vi "qr.vi"(9 "stop":bool, 11 "Session In":T2) -> (1 "Image":T1(plugin-control), 2 "Found?":bool, 3 "Data":string)   [LabVIEW 2019]
uses:
  <vilib>/userdefined/High Color/IMAQdx.ctl
  <vilib>/vision/driver/NI_Vision_Acquisition_Software.lvlib
  <vilib>/vision/NI_Vision_Development_Module.lvlib
panel:
  out "error out 2":errorcluster
  out "error out 3":errorcluster
  out "error out":errorcluster
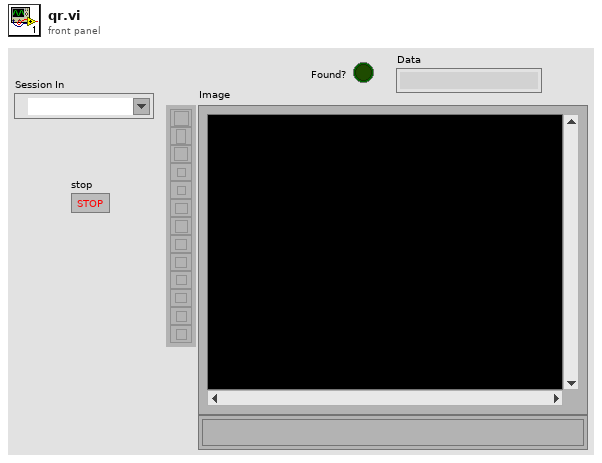
[diagram p1: front panel]
types:
  T1 = typedef "IMAQ Image.ctl" = refnum<image>
  T2 = typedef "IMAQdx.ctl" = refnum<k21>
  T3 = typedef "Image Type" = u32
  T4 = typedef "QR Code Report.ctl" = cluster{"Found?":bool, "Data":string, "Bounding Box":cluster{"x":sgl, "y":sgl}[], "Errors Corrected":u32, "Dimensions (Rows/Cols)":u32, "Version":u32, "QR Model":T5, "Stream Mode":T6, "Barcode Polarity":T7, "Mirrored?":bool, "Append Stream Position":u32, "Size of Append Stream":u32, "First EAN-128 ID":i32, "First Alternate Language ID":i32, "Append Stream ID":u32, "Minimum Edge Strength":u32, "Demodulation Mode":T8, "Cell Sample Size":T9, "Cell Filter Mode":T10}
  T5 = typedef "QR Code Model Type.ctl" = i32
  T6 = typedef "QR Code Stream Mode Type.ctl" = i32
  T7 = typedef "Data Matrix Polarity.ctl" = i32
  T8 = typedef "Demodulation Mode.ctl" = i32
  T9 = typedef "Cell Sample Size.ctl" = i32
  T10 = typedef "Cell Filter Mode.ctl" = i32
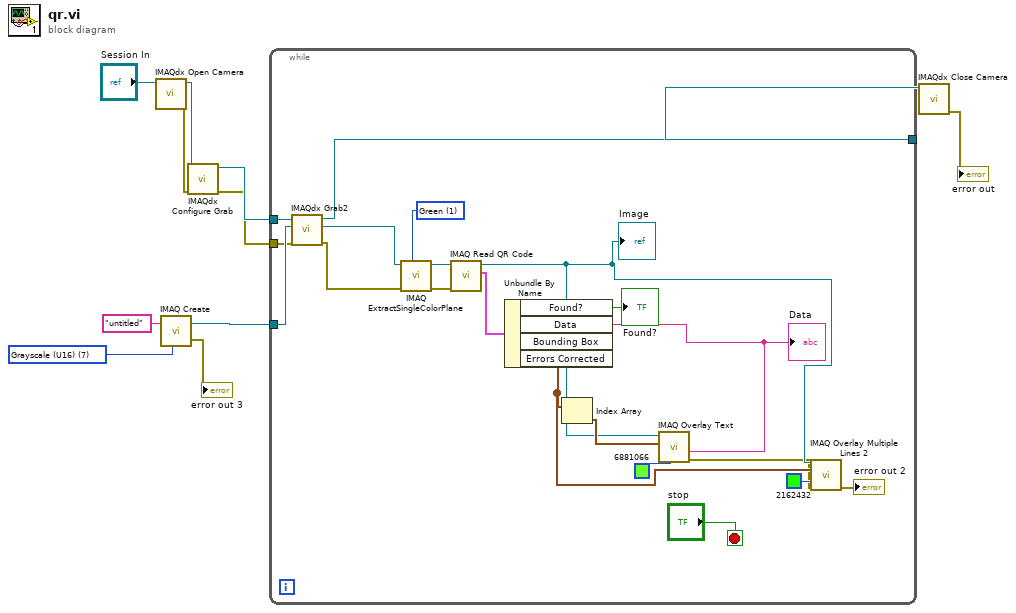
[diagram p0: block diagram]
diagram:
  w1 = T3 7 items=["Grayscale (U8)", "Grayscale (I16)", "Grayscale (SGL)", "Complex (CSG)", "RGB (U32)", "HSL (U32)", "RGB (U64)", "Grayscale (U16)"] ("Image Type")
  n1 = call <vilib>:"IMAQdx Open Camera.vi"("Session In"="Session In") -> ("error out"=w9:errorcluster, "Session Out"=w10:T2)  [unwired: 9 in]
  n2 = call "IMAQ Create"("Image Name"="untitled", "Image Type"=w1) -> ("New Image"=w6:T1, "error out"=→"error out 3":errorcluster)  [unwired: 3 in]
  n3 = call <vilib>:"IMAQdx Configure Grab.vi"("error in"=w9, "Session In"=w10) -> ("error out"=w3:errorcluster, "Session Out"=w7:T2)  [unwired: 8 in]
  n4 = while {
    tunnel: w7 -> [w30]
    tunnel: w6 -> [w31]
    tunnel: [w23] -> w4
    tunnel: w3 -> [w28]
    stop <- "stop" stop-if-true
    w22 = 1 items=["Red", "Green", "Blue", "Hue", "Saturation", "Luminance", "Value", "Intensity"] ("Color Plane")
    n5 = call <vilib>:"IMAQdx Grab2.vi"("error in"=w28, "Image In"=w31, "Session In"=w30) -> ("error out"=w25:errorcluster, "Image Out"=w24:T1, "Session Out"=w23:T2)  [unwired: 5 in, 1 out]
    n6 = call "IMAQ ExtractSingleColorPlane"("Color Plane"=w22, "error in (no error)"=w25, "Image Src"=w24) -> ("error out"=w27:errorcluster, "Image Dst Out"=w26:T1)  [unwired: 7 in]
    n7 = call "IMAQ Read QR Code"("error in (no error)"=w27, "Image"=w26) -> ("QR Code Report"=w21:T4, "Image (duplicate)"=w16:T1)  [unwired: 6 in, 2 out]
    "Image" <- w16
    n8 = Unbundle By Name(w21) -> ("Found?"=→"Found?":bool, "Data"=w18:string, "Bounding Box"=w15:cluster{"x":sgl, "y":sgl}[])  [unwired: 1 out]
    "Data" <- w18
    n9 = Index Array(array=w15) -> (element=w19:cluster{"x":sgl, "y":sgl})  [unwired: 1 in]
    n10 = call "IMAQ Overlay Text"("Text Color (black)"=u32 6881066, "String"=w18, "Origin"=w19, "Image"=w16) -> ("error out"=w13:errorcluster)  [unwired: 6 in, 1 out]
    n11 = call "IMAQ Overlay Multiple Lines 2"("Image"=w16, "Line End Points"=w15, "Color"=u32 2162432, "error in (no error)"=w13) -> ("error out"=→"error out 2":errorcluster)  [unwired: 10 in, 1 out]
  }
  n12 = call <vilib>:"IMAQdx Close Camera.vi"("Session In"=w4) -> ("error out"=→"error out":errorcluster)  [unwired: 10 in]
